vi "Convert Binary file to Text.vi"(6 "Text format":T1, 7 "Originating directory":path, 8 "error in (no error)":errorcluster, 10 "NCL File Path":path, 11 "Destination directory":path) -> (0 "error out":errorcluster)   [LabVIEW 2010, in "CAN Log Transfer and Convert.lvlib"]
uses:
  CAN Log Transfer and Convert.lvlib
  Text Format.ctl
  Display NCL Logfile as CAN Frames Folder/logfile.llb/XNET Logfile Mode.ctl
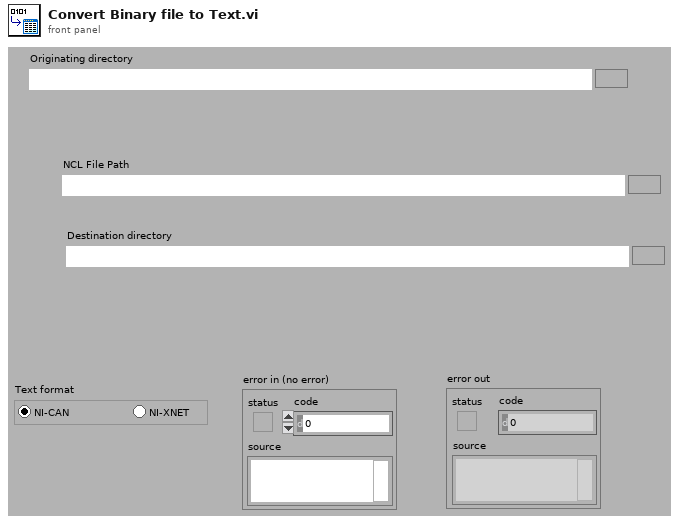
[diagram p1: front panel]
types:
  T1 = typedef "CAN Log Transfer and Convert.lvlib/Text Format.ctl" = enum32{"NI-CAN", "NI-XNET"}
  T2 = typedef "XNET Logfile Mode.ctl" = enum16{"Read", "Write (native endian)", "Write (big endian)"}
  T3 = typedef "XNET Logfile.ctl" = cluster{" file refnum":refnum<file>, "endian swap?":bool, "partial":u8[]}
  T4 = typedef "XNET Frame CAN.ctl" = cluster{"timestamp":timestamp, "payload":u8[], "identifier":u32, "type":T5, "extended?":bool, "echo?":bool}
  T5 = typedef "XNET Frame Type CAN.ctl" = u8
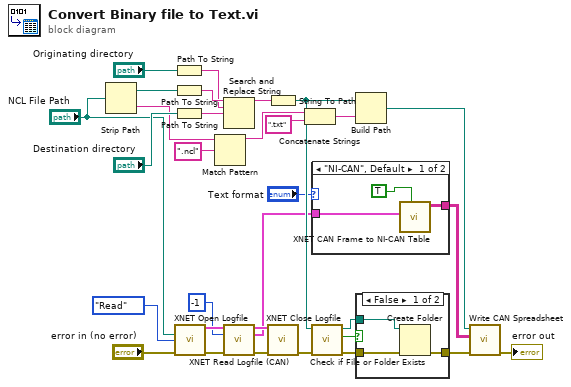
[diagram p0: block diagram]
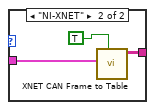
[diagram p2: hidden frame]
diagram:
  n1 = Strip Path(path="NCL File Path") -> (stripped path=w13:path, name=w18:string)
  n2 = Path To String(path="Originating directory") -> (string=w26:string)
  n3 = Path To String(path=w13) -> (string=w27:string)
  n4 = Path To String(path="Destination directory") -> (string=w25:string)
  n5 = call "XNET Open Logfile.vi"("filepath"="NCL File Path", "mode"=XNET_Logfile_Mode."Read", "error in"="error in (no error)") -> ("logfile out"=w11:T3, "error out"=w10:errorcluster)  [unwired: 11 in]
  n6 = Match Pattern(string=w18, regular expression=".ncl") -> (before substring=w17:string)  [unwired: 1 in, 3 out]
  n7 = Search and Replace String(input string=w27, search string=w26, replace string=w25) -> (result string=w24:string)  [unwired: 5 in, 3 out]
  n8 = call "XNET Read Logfile (CAN).vi"("logfile in"=w11, "Maximum Number of Frames to read"=-1 ("Number of Frames to read (-1:all)"), "error in"=w10) -> ("logfile out"=w8:T3, "CAN frames"=w7:T4[], "error out"=w9:errorcluster)  [unwired: 8 in, 2 out]
  n9 = String To Path(string=w24) -> (path=w23:path)
  n10 = call "XNET Close Logfile.vi"("logfile  in"=w8, "error in"=w9) -> ("error out"=w3:errorcluster)  [unwired: 12 in, 1 out]
  n11 = Concatenate Strings(w17, ".txt" ("string")) -> (w30:string)
  n12 = case shown="\"NI-CAN\", Default" "Text format" {
    tunnel: w7 -> [w34 w37]
    tunnel: [w32 w35] -> w1
    frame "NI-CAN", Default {
      n13 = call "XNET CAN Frame to NI-CAN Table.vi"("Hexadecimal?"=TRUE, "CAN Frames (from XNET Read)"=w34) -> ("Output Array"=w32:string[][])  [unwired: 9 in]
    }
    frame "NI-XNET" {
      n14 = call "XNET CAN Frame to Table.vi"("Hexadecimal?"=TRUE, "CAN Frames (from XNET Read)"=w37) -> ("Output Array"=w35:string[][])  [unwired: 9 in]
    }
  }
  n15 = call <vilib>:"Check if File or Folder Exists.vi"("error in (no error)"=w3, "path"=w23) -> ("error out"=w21:errorcluster, "file or folder exists?"=w20:bool, "dup path"=w22:path)  [unwired: 7 in]
  n16 = Build Path(base path=w23, name or relative path=w30) -> (appended path=w14:path)
  n17 = case shown="False" w20 {
    tunnel: [w40 w41] -> w16
    tunnel: w22 -> [w39 _]
    tunnel: w21 -> [w38 w41]
    frame False {
      n18 = Create Folder(path (use dialog)=w39, error in=w38) -> (error out=w40:errorcluster)  [unwired: 1 in, 2 out]
    }
    frame True {
    }
  }
  n19 = call "Write CAN Spreadsheet.vi"("error in"=w16, "2D data"=w1, "file path"=w14) -> ("error out"=→"error out":errorcluster)  [unwired: 7 in, 1 out]
